vi "Live window-Channel ctrls state.vi"() -> ()   [LabVIEW 2017]
uses:
  Typedefs/Channel control synergistic behaviour enum.ctl
panel:
  out "error out":errorcluster
  in  "error in (no error)":errorcluster
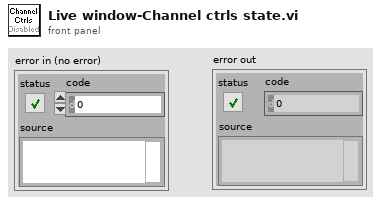
[diagram p1: front panel]
types:
  T1 = typedef "Channel control synergistic behaviour enum.ctl" = enum16{"Left disabled-Right enabled", "Left enabled-Right disabled", "Both enabled"}
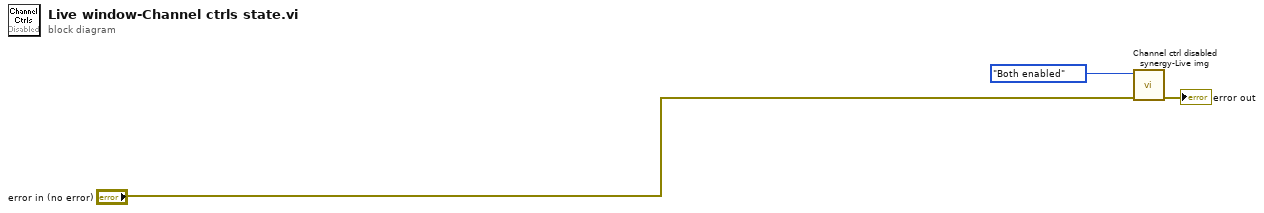
[diagram p0: block diagram]
diagram:
  n1 = call "Channel ctrl disabled synergy-Live img.vi"("error in (no error)"="error in (no error)", "Behaviour"=Channel_control_synergistic_behaviour_enum."Both enabled") -> ("error out"=→"error out":errorcluster)  [unwired: 9 in]
